vi "UDPSendData.vi"(8 "error in (no error)":errorcluster, 11 "connection ID":refnum<k16>) -> ()   [LabVIEW 2015]
uses:
  VisionGlobals.vi
  GlobalVisionVars.vi
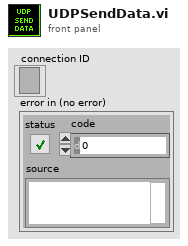
[diagram p1: front panel]
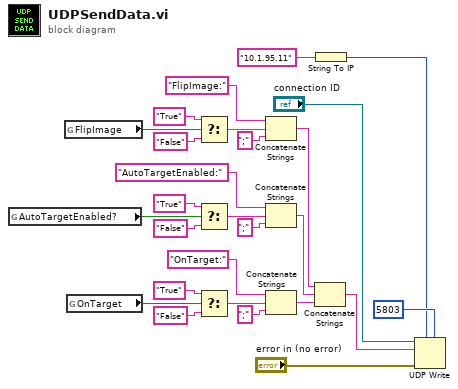
[diagram p0: block diagram]
diagram:
  n1 = global read "VisionGlobals.vi" "AutoTargetEnabled?"() -> (w1:bool)
  n2 = global read "VisionGlobals.vi" "FlipImage"() -> (w22:bool)
  n3 = global read "GlobalVisionVars.vi" "OnTarget"() -> (w2:bool)
  n4 = Select(t="True", s=w22, f="False") -> (s? t:f=w18:string)
  n5 = Select(t="True", s=w1, f="False") -> (s? t:f=w13:string)
  n6 = Select(t="True", s=w2, f="False") -> (s? t:f=w8:string)
  n7 = Concatenate Strings("FlipImage:", w18, ";" ("string")) -> (w6:string)
  n8 = Concatenate Strings("AutoTargetEnabled:", w13, ";" ("string")) -> (w5:string)
  n9 = Concatenate Strings("OnTarget:", w8, ";" ("string")) -> (w4:string)
  n10 = Concatenate Strings(w6, w5, w4) -> (w3:string)
  n11 = String To IP(1:"10.1.95.11" ("name")) -> (0:w24:u32)
  n12 = UDP Write(address=w24, port or service name=u16 5803, connection ID="connection ID", data in=w3, 8:"error in (no error)") -> ()  [unwired: 1 in, 2 out]
